vi "9068_Main.vi"() -> ()   [LabVIEW 2014]
doc: "This application launches and executes the Tag Bus Data framework configuration for the specified target alias. This is a simple example of the framework API functions, but may also be a suitable starting point for a Host UI or Thick Client that is running a local version of the framework."
uses:
  <vilib>/NI/Module Execution Interface/Engine Runtime/Execution States.ctl
  <vilib>/NI/Module Execution Interface/Engine Runtime/Fault.ctl
  <vilib>/NI/Tag Bus Module Framework/runtime/error classification.ctl
  <vilib>/userdefined/High Color/nirio_resource_hc.ctl
  <vilib>/NI/Module Execution Interface/Engine Runtime/Engine Runtime Interface.lvclass
  <vilib>/NI/DCAF/Tag Editor Core/Framework Configuration Classes/target runtime/PL_Target Runtime.lvclass
  <vilib>/NI/Tag Bus Module Framework/FPGA manager/FPGA manager.lvlib
  <vilib>/rvi/interface/nirviOpenFPGA/nirviOpenFPGA.xnode
  <vilib>/NI/Tag Bus Module Framework/FPGA manager/methods.ctl
  <vilib>/NI/Tag Bus Module Framework/runtime/TBM module execution interface.lvclass
panel:
  out "error out":errorcluster
  in  "error in (no error)":errorcluster
  in  "run time":u32=5
  in  "configuration file path":path=path "/home/lvuser/Endurance_Testing_Configuration.pcfg"
  in  "target alias":string="cRIO9068"
  out "engine status":T4(array[cluster])
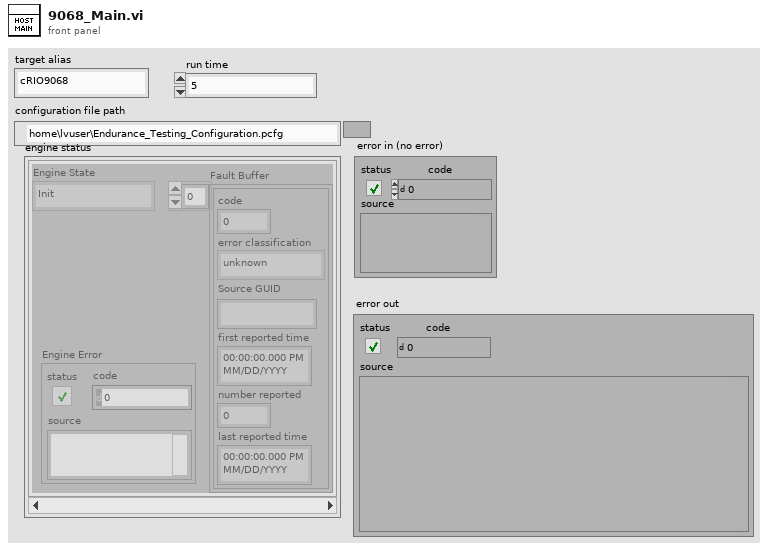
[diagram p1: front panel]
types:
  T1 = typedef "Engine Runtime Interface.lvclass/Execution States.ctl" = enum16{"Init", "Pre-Operational", "Safe-Operational", "Operational", "Stopped"}
  T2 = typedef "Engine Runtime Interface.lvclass/Fault.ctl" = cluster{"code":i32, "error classification":T3, "Source GUID":string, "first reported time":timestamp, "number reported":u32, "last reported time":timestamp}
  T3 = typedef "TBM module execution interface.lvclass/error classification.ctl" = enum16{"unknown", "none", "trivial", "recoverable", "critical"}
  T4 = cluster{"Engine State":T1, "Fault Buffer":T2[], "Engine Error":errorcluster}[]
  T5 = typedef "FPGA manager.lvlib/methods.ctl" = enum16{"initialize bitfile", "cache bitfile", "locate bitfile", "close bitfile", "clear manager"}
  T6 = typedef "nirio_resource_hc.ctl" = tag
  T7 = cluster{"Engine State":T1, "faults":T2[], "Engine Error":errorcluster}
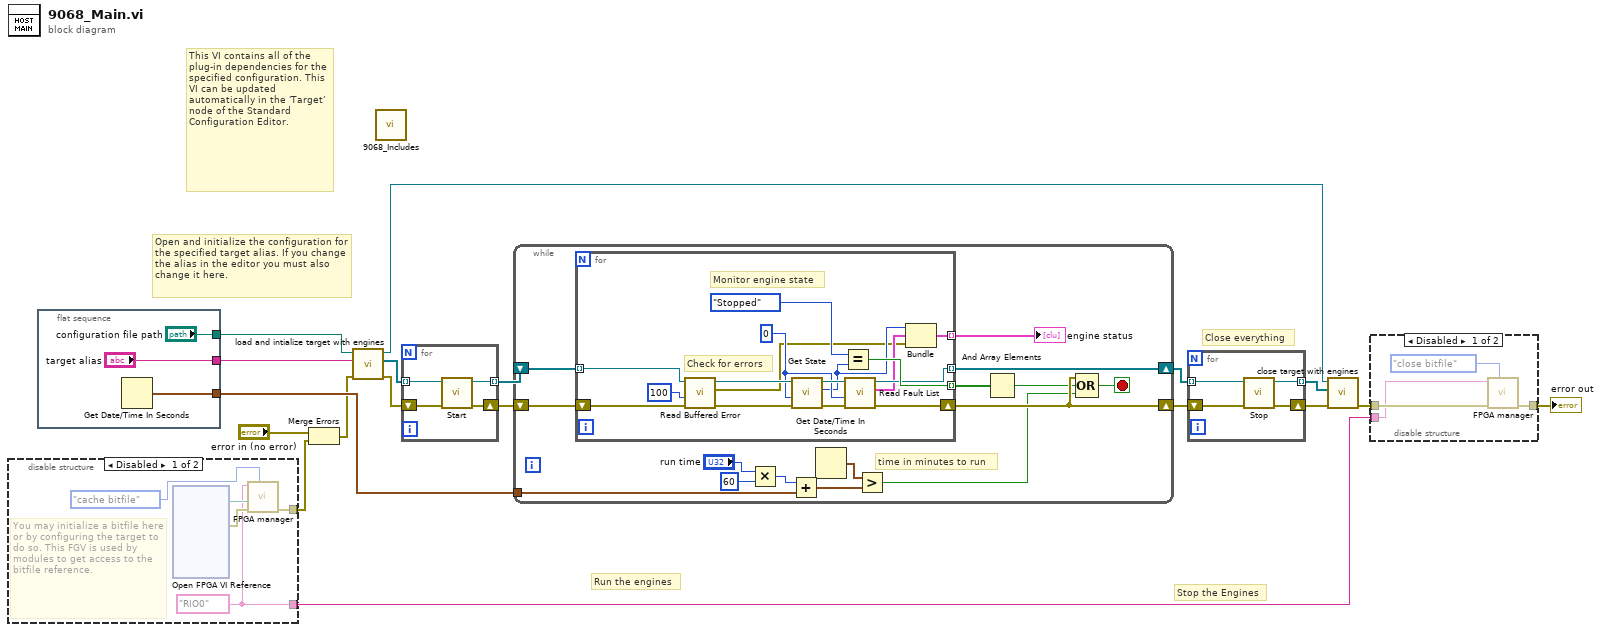
[diagram p0: block diagram]
diagram:
  # "Open and initialize the configuration for the specified target alias. If you change the alias in the editor you must also change it here."
  # "Close everything"
  # "Stop the Engines"
  # "This VI contains all of the plug-in dependencies for the specified configuration. This VI can be updated automatically in the 'Target' node of the Standard Configuration Editor."
  # "Run the engines"
  n1 = disable-structure shown="Disabled" {
    disable-tunnel: [w23 _] -> w3
    disable-tunnel: [w19 _] -> w5
    frame Disabled {
      w19 = T6 "RIO0" ("RIO resource")
      # "You may initialize a bitfile here or by configuring the target to do so. This FGV is used by modules to get access to the bitfile reference."
      n2 = xnode "Open FPGA VI Reference"() -> ("FPGA VI Reference Out"=w21:refnum<k20>, "error out"=w22:errorcluster)  [unwired: 2 in]
      n3 = call <vilib>:"FPGA manager.vi"("action"=methods."cache bitfile", "error in"=w22, "bitfile to cache"=w21, "RIO resource"=w19) -> ("error out"=w23:errorcluster)  [unwired: 5 in, 2 out]
    }
    frame Enabled {
    }
  }
  n4 = flat-sequence {
    tunnel: ["target alias"] -> w13
    tunnel: ["configuration file path"] -> w9
    tunnel: [w24] -> w6
    frame #0 {
      n5 = Get Date/Time In Seconds() -> (seconds since 1Jan1904=w24:timestamp)
    }
  }
  n6 = Merge Errors("error in (no error)", w3) -> (w2:errorcluster)
  n7 = call <vilib>:"load and intialize target with engines.vi"("error in"=w2, "target alias"=w13, "file path"=w9) -> ("error out"=w15:errorcluster, "engine runtime interfaces"=w14:refnum<class "Engine Runtime Interface.lvclass">[], "target runtime"=w11:refnum<class "PL_Target Runtime.lvclass">)  [unwired: 6 in]
  n8 = call "9068_Includes.vi"() -> ()  [unwired: 12 in]
  n9 = for {
    tunnel: [w30] -> w18 mode=indexing
    tunnel: w14 -> [w27] mode=indexing
    shift-right: [w29] -> w7
    shift-left: w15 -> [w28]
    n10 = call-dynamic "Start.vi"("error in"=w28, "Engine Runtime Interface in"=w27) -> ("error out"=w29:errorcluster, "Engine Runtime Interface out"=w30:refnum<class "Engine Runtime Interface.lvclass">)  [unwired: 8 in]
  }
  n11 = while {
    shift-right: [w43] -> w17
    shift-left: w18 -> [w45]
    shift-right: [w41] -> w16
    shift-left: w7 -> [w44]
    tunnel: w6 -> [w35]
    stop <- w42 stop-if-true
    # "time in minutes to run"
    n12 = for {
      tunnel: w45 -> [w61] mode=indexing
      tunnel: [w52] -> w43 mode=indexing
      tunnel: [w56] -> w39 mode=indexing
      shift-right: [w51] -> w41
      shift-left: w44 -> [w60]
      tunnel: [w46] -> w40 mode=indexing
      w50 = 0 ("timeout (-1)")
      # "Monitor engine state"
      # "Check for errors"
      n13 = call-dynamic "Read Buffered Error.vi"("error in"=w60, "timeout in ms (0)"=100, "Engine Runtime Interface in"=w61) -> ("error out"=w58:errorcluster, "Engine Error"=w47:errorcluster, "Engine Runtime Interface out"=w59:refnum<class "Engine Runtime Interface.lvclass">)  [unwired: 6 in]
      n14 = call-dynamic "Get State.vi"("error in"=w58, "timeout (-1)"=w50, "Engine Runtime Interface in"=w59) -> ("error out"=w54:errorcluster, "Engine State"=w49:T1, "Engine Runtime Interface out"=w53:refnum<class "Engine Runtime Interface.lvclass">)  [unwired: 6 in]
      n15 = Equal?(x=Execution_States."Stopped" ("Engine State"), y=w49) -> (x = y?=w56:bool)
      n16 = call-dynamic "Read Fault List.vi"("error in"=w54, "timeout (-1)"=w50, "Engine Runtime Interface in"=w53) -> ("error out"=w51:errorcluster, "faults"=w48:T2[], "Engine Runtime Interface out"=w52:refnum<class "Engine Runtime Interface.lvclass">)  [unwired: 6 in]
      n17 = Bundle("Engine State"=w49, "faults"=w48, "Engine Error"=w47) -> (w46:T7)  [unwired: 1 in]
    }
    "engine status" <- w40
    n18 = Multiply(x="run time", y=u32 60) -> (x*y=w33:u32)
    n19 = Add(x=w33, y=w35) -> (x+y=w37:timestamp)
    n20 = Get Date/Time In Seconds() -> (seconds since 1Jan1904=w34:timestamp)
    n21 = Greater?(x=w34, y=w37) -> (0:w36:bool)
    n22 = And Array Elements(Boolean array=w39) -> (logical AND=w38:bool)
    n23 = Compound Arithmetic op=OR(w41, w38, w36) -> (w42:bool)
  }
  n24 = for {
    tunnel: w17 -> [w65] mode=indexing
    shift-right: [w62] -> w10
    shift-left: w16 -> [w64]
    tunnel: [w63] -> w12 mode=indexing
    n25 = call-dynamic "Stop.vi"("error in"=w64, "Engine Runtime Interface in"=w65) -> ("error out"=w62:errorcluster, "Engine Runtime Interface out"=w63:refnum<class "Engine Runtime Interface.lvclass">)  [unwired: 8 in]
  }
  n26 = call <vilib>:"close target with engines.vi"("error in"=w10, "Engine Runtime Interfaces"=w12, "Target Runtime"=w11) -> ("error out"=w8:errorcluster)  [unwired: 8 in]
  n27 = disable-structure shown="Disabled" {
    disable-tunnel: [w68 w70] -> w1
    disable-tunnel: w8 -> [w69 w70]
    disable-tunnel: w5 -> [w66 _]
    frame Disabled {
      n28 = call <vilib>:"FPGA manager.vi"("action"=methods."close bitfile", "error in"=w69, "RIO resource"=w66) -> ("error out"=w68:errorcluster)  [unwired: 6 in, 2 out]
    }
    frame Enabled {
    }
  }
  "error out" <- w1
